vi "Agilent N934X Series Acquire Trace.vi"() -> ()   [LabVIEW 2022 SP3]
doc: "This example shows how to configure the spectrum analyzer to acquire a trace."
uses:
  <instrlib>/Agilent N934X Series/Agilent N934X Series.lvlib
panel:
  out "Trace Waveform":T1(graph)
  in  "Timeout (10000ms)":i32=10000
  in  "Amplitude Units (0: dBm)":i32(ring) items=["dBm", "dBmV", "dBmVEMF", "dBuV", "dBuVEMF", "V", "W", "VEMF"]
  in  "Reference Level Offset (0 dB)":dbl
  in  "Reference Level (0 dBm)":i32
  in  "Stop Frequency (7 GHz)":dbl=7000000000.0
  in  "Start Frequency (0)":dbl
  in  "VISA resource name":refnum<visa-resource-name>
  # "(c) 2012 - 2025 National Instruments.  ALL RIGHTS RESERVED."
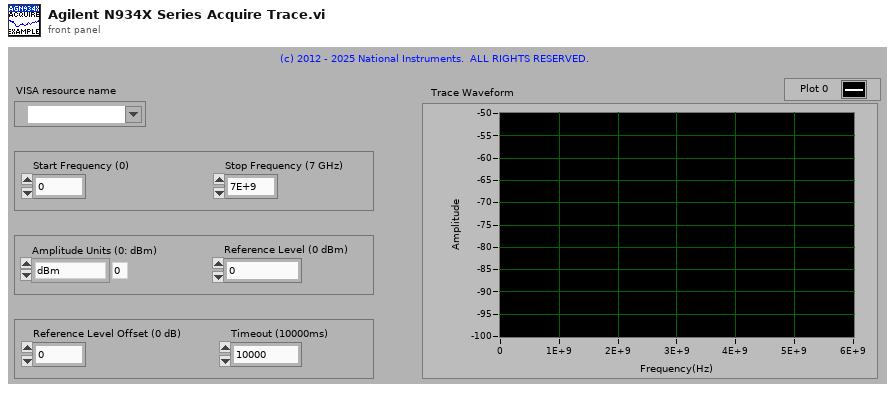
[diagram p1: front panel]
types:
  T1 = cluster{"Start Frequency (0)":dbl, dbl, "Trace Data":dbl[]}
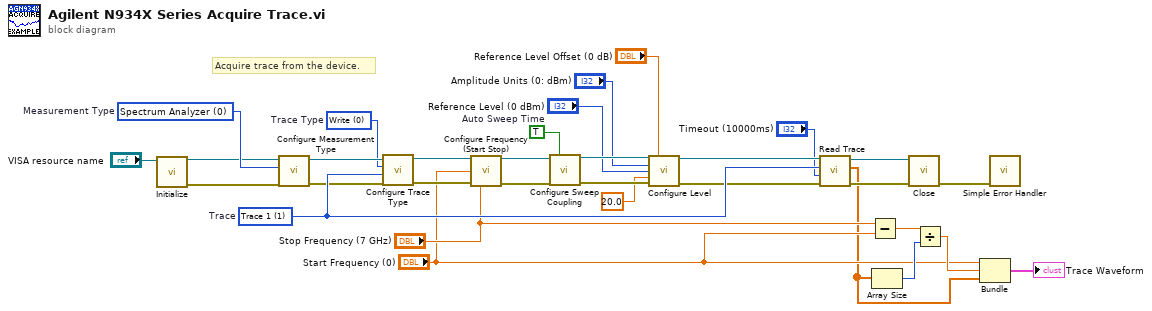
[diagram p0: block diagram]
diagram:
  w6 = TRUE  # Auto Sweep Time
  w25 = 1 items=["Trace 1"=1, "Trace 2"=2, "Trace 3"=3, "Trace 4"=4]  # Trace
  w28 = 0 items=["Write", "Maximum hold", "Minimum hold", "View", "Blank"]  # Trace Type
  w31 = 0 items=["Spectrum Analyzer", "Tracking Generator", "Power Meter"]  # Measurement Type
  # "Acquire trace from the device."
  n1 = call <instrlib>:"Initialize.vi"("VISA resource name"="VISA resource name") -> ("error out"=w21:errorcluster, "VISA resource name out"=w30:refnum<visa-resource-name>)  [unwired: 9 in]
  n2 = call <instrlib>:"Configure Measurement Type.vi"("error in (no error)"=w21, "Measurement Type (0: Spectrum Analyzer)"=w31, "VISA resource name"=w30) -> ("error out"=w20:errorcluster, "VISA resource name out"=w29:refnum<visa-resource-name>)  [unwired: 7 in]
  n3 = call <instrlib>:"Configure Trace Type.vi"("error in (no error)"=w20, "Trace (1: Trace 1)"=w25, "Trace Type (0: Write)"=w28, "VISA resource name"=w29) -> ("error out"=w19:errorcluster, "VISA resource name out"=w27:refnum<visa-resource-name>)  [unwired: 6 in]
  n4 = call <instrlib>:"Configure Frequency (Start Stop).vi"("VISA resource name"=w27, "Start Frequency (9E+3 Hz)"="Start Frequency (0)", "error in (no error)"=w19, "Stop Frequency (7E+9 Hz)"="Stop Frequency (7 GHz)") -> ("VISA resource name out"=w10:refnum<visa-resource-name>, "error out"=w9:errorcluster)  [unwired: 10 in]
  n5 = call <instrlib>:"Configure Sweep Coupling.vi"("VISA resource name"=w10, "Auto Sweep Time (T: Enable)"=w6, "error in (no error)"=w9) -> ("VISA resource name out"=w7:refnum<visa-resource-name>, "error out"=w8:errorcluster)  [unwired: 11 in]
  n6 = call <instrlib>:"Configure Level.vi"("VISA resource name"=w7, "Reference Level Offset (0 dB)"="Reference Level Offset (0 dB)", "Amplitude Units (0: dBm)"="Amplitude Units (0: dBm)", "Reference Level (0 dBm)"="Reference Level (0 dBm)", "Manual Attenuation (20 dB)"=20.0, "error in (no error)"=w8) -> ("VISA resource name out"=w26:refnum<visa-resource-name>, "error out"=w18:errorcluster)  [unwired: 8 in]
  n7 = call <instrlib>:"Read Trace.vi"("error in (no error)"=w18, "Timeout (10000ms)"="Timeout (10000ms)", "Trace (1: Trace 1)"=w25, "VISA resource name"=w26) -> ("error out"=w17:errorcluster, "Trace Data"=w2:dbl[], "VISA resource name out"=w22:refnum<visa-resource-name>)  [unwired: 5 in]
  n8 = Subtract(x="Stop Frequency (7 GHz)", y="Start Frequency (0)") -> (x-y=w15:dbl)
  n9 = Array Size(array=w2) -> (size(s)=w14:i32)
  n10 = call <instrlib>:"Close.vi"("error in (no error)"=w17, "VISA resource name"=w22) -> ("error out"=w23:errorcluster)  [unwired: 9 in]
  n11 = Divide(x=w15, y=w14) -> (x/y=w13:dbl)
  n12 = Bundle("Start Frequency (0)"="Start Frequency (0)", w13, "Trace Data"=w2) -> (→"Trace Waveform":T1)  [unwired: 1 in]
  n13 = call <vilib>:"Simple Error Handler.vi"("error in (no error)"=w23) -> ()  [unwired: 4 in, 5 out]
